vi "1B_AmplitudeRampResults.vi"(7 "Tolerance [ A ]":dbl=0.0009 format="%#.3p", 9 "Array 2":T1(array[cluster]), 10 "Time":dbl[](array[numeric]), 11 "Array 3":dbl[][](array[numeric])) -> (0 "Cluster 2":cluster{dbl[], dbl[]}, 1 "Array":T2(array[cluster]), 2 "Cluster 3":cluster{dbl[], dbl[]}, 3 "Cluster 4":cluster{dbl[], dbl[]}, 4 "Cluster":cluster{dbl[], dbl[]}, 5 "P1 mean error [ A ]":dbl format="%#.0p", 8 "Measured Frequency":dbl[](array[numeric]) format="%#.1p")   [LabVIEW 2010]
panel:
  out "measured time offset (sec )":dbl format="%#.1p"
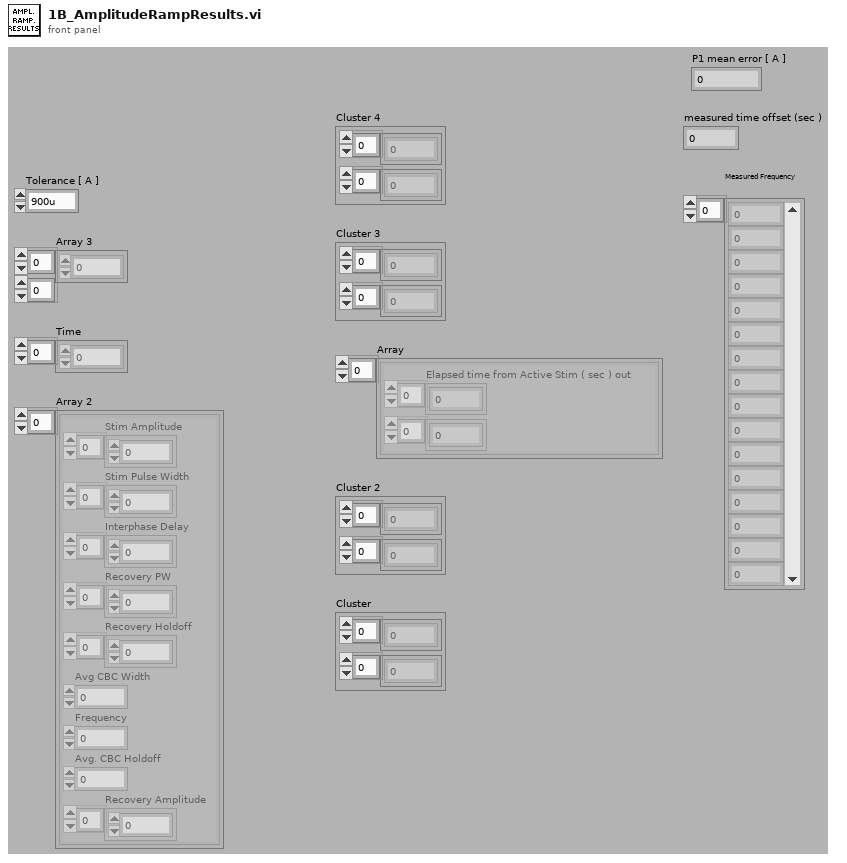
[diagram p1: front panel]
types:
  T1 = cluster{"Stim Amplitude":dbl[], "Stim Pulse Width":dbl[], "Interphase Delay":dbl[], "Recovery PW":dbl[], "Recovery Holdoff":dbl[], "Avg CBC Width":dbl, "Frequency":dbl, "Avg. CBC Holdoff":dbl, "Recovery Amplitude":dbl[]}[]
  T2 = cluster{"Elapsed time from Active Stim ( sec ) out":dbl[], dbl[]}[]
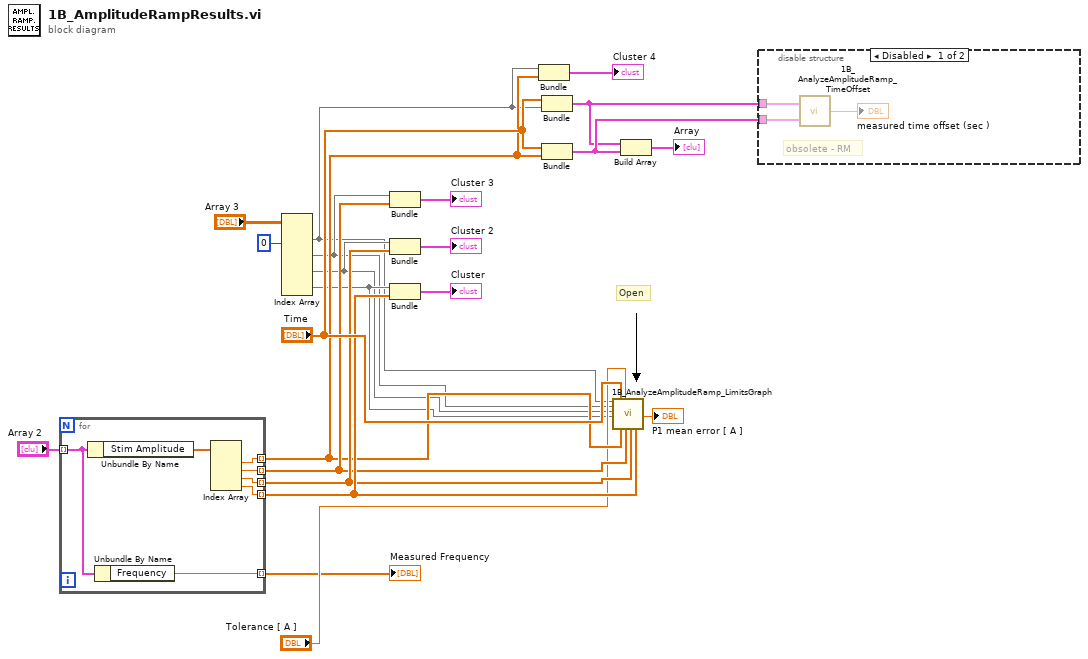
[diagram p0: block diagram]
diagram:
  # "Open"
  n1 = for {
    tunnel: "Array 2" -> [w27] mode=indexing
    tunnel: [w28] -> w18 mode=indexing
    tunnel: [w26] -> w5 mode=indexing
    tunnel: [w25] -> w19 mode=indexing
    tunnel: [w24] -> w20 mode=indexing
    tunnel: [w23] -> w21 mode=indexing
    n2 = Unbundle By Name(w27) -> ("Stim Amplitude"=w29:dbl[])
    n3 = Unbundle By Name(w27) -> ("Frequency"=w26:dbl)
    n4 = Index Array(array=w29) -> (element #1=w28:dbl, element #2=w25:dbl, element #3=w24:dbl, element #4=w23:dbl)  [unwired: 4 in]
  }
  "Measured Frequency" <- w5
  n5 = Index Array(array="Array 3", index (col) #1=0 ("disabled index (col)")) -> (element #1=w13:dbl[], element #2=w14:dbl[], element #3=w15:dbl[], element #4=w16:dbl[])  [unwired: 7 in]
  n6 = Bundle("Array 3"=w14, w19) -> (→"Cluster 3":cluster{"Array 3":dbl[], dbl[]})  [unwired: 1 in]
  n7 = Bundle("Array 3"=w15, w20) -> (→"Cluster 2":cluster{"Array 3":dbl[], dbl[]})  [unwired: 1 in]
  n8 = Bundle("Array 3"=w16, w21) -> (→"Cluster":cluster{"Array 3":dbl[], dbl[]})  [unwired: 1 in]
  n9 = Bundle("Array 3"=w13, w18) -> (→"Cluster 4":cluster{"Array 3":dbl[], dbl[]})  [unwired: 1 in]
  n10 = Bundle("Time"="Time", "Array 3"=w13) -> (w6:cluster{"Time":dbl[], "Array 3":dbl[]})  [unwired: 1 in]
  n11 = Bundle("Time"="Time", w18) -> (w7:cluster{"Time":dbl[], dbl[]})  [unwired: 1 in]
  n12 = call "1B_AnalyzeAmplitudeRamp_LimitsGraph.vi"("Target P1"=w13, "Target P2"=w14, "Target P3"=w15, "Target P4"=w16, "Trimmed Elapsed time from Active Stim ( sec )"="Time", "Meas. P 1"=w18, "Tol [ A ]"="Tolerance [ A ]", "Meas. P 2"=w19, "Meas. P 3"=w20, "Meas. P 4"=w21) -> ("P1 mean error [ A ]"=→"P1 mean error [ A ]":dbl)  [unwired: 9 in]
  n13 = Build Array(w6, w7) -> (→"Array":cluster{"Time":dbl[], "Array 3":dbl[]}[])
  n14 = disable-structure shown="Disabled" {
    disable-tunnel: w7 -> [w31 _]
    disable-tunnel: w6 -> [w30 _]
    frame Disabled {
      # "obsolete - RM"
      n15 = call "1B_AnalyzeAmplitudeRamp_TimeOffset.vi"("Measured"=w31, "Target"=w30) -> ("delta x for the same Y ( time offset )"=→"measured time offset (sec )":dbl)
    }
    frame Enabled {
    }
  }
